vi "Get Shortest Distance Preference.vi"() -> (0 "Use Shortest Distance Relative? Out":bool)   [LabVIEW 2011, in "Pivot Drive.lvlib"]
doc: "Gets wether or not to use shortest distance relative or absolute in the pivot system.\nShortest Distance Relative (a true value)\nReturns a value that is either the smallest angle between the current and wanted values or the conterminal of the current and the regular of the wanted values.\nWhichever is smaller.\nIf the conterminal of the current is matched with the regular of the wanted then the drive motors are flipped (I.E. 0 Wanted and 180 current will negate the drive motor.)\nHas a domain of -90 to 90 degrees.\nShortest Distance Absolute (A false value)\nReturns a value that is the angle between the current and wanted angles.\nDoes not negate the drive wheels.\nIf the wheel is at 0 degrees but the setpoint is 180 degrees the wheel will spin all the way to 180 degrees.\nHas a domain of -180 and 180 degrees."
uses:
  Pivot Drive.lvlib
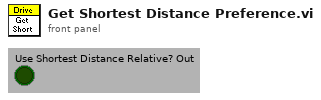
[diagram p1: front panel]
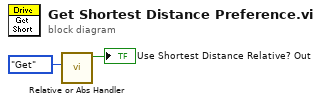
[diagram p0: block diagram]
diagram:
  n1 = call "Relative or Abs Handler.vi"("Set or Get"=enum16{"Set", "Get"}."Get") -> ("Use Shortest Distance Relative? Out"=→"Use Shortest Distance Relative? Out":bool)  [unwired: 1 in, 9 out]
